vi "AddBandstoBandNames.vi"(11 "filter name":string) -> (1 "File Name":string[](array[string]), 3 "Extended Name":string[](array[string]))   [LabVIEW 2022 SP3]
uses:
  <vilib>/Utility/error.llb/whitespace.ctl
  <vilib>/Utility/error.llb/Trim Whitespace One-Sided.vi
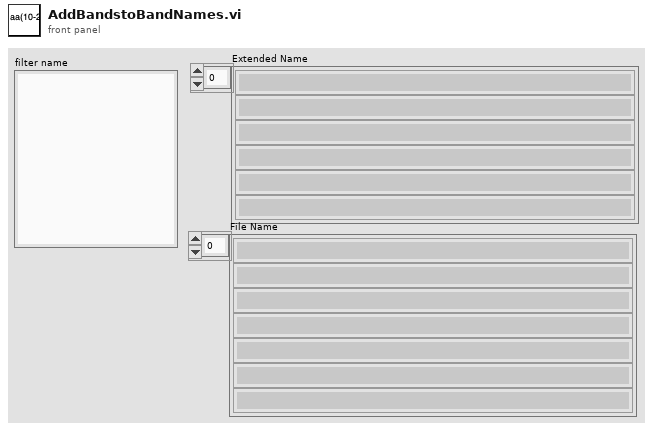
[diagram p1: front panel]
types:
  T1 = typedef "whitespace.ctl" = u16
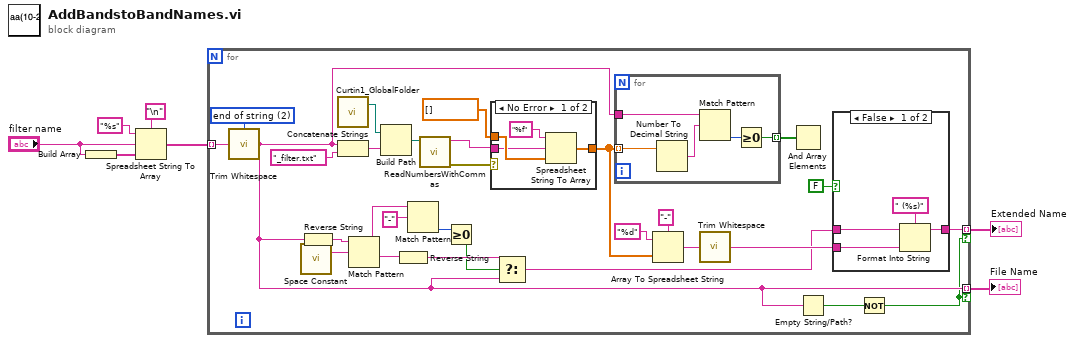
[diagram p0: block diagram]
diagram:
  n1 = Build Array("filter name") -> (w5:string[])
  n2 = Spreadsheet String To Array(delimiter (Tab)="\n" ("format string"), format string="%s", spreadsheet string="filter name", array type (2D Dbl)=w5) -> (array=w4:string[])
  n3 = for {
    tunnel: w4 -> [w25] mode=indexing
    tunnel: [w29] -> w3 mode=indexing if=w14
    tunnel: [w16] -> w2 mode=indexing if=w14
    w11 = T1 2 items=["both", "start of string", "end of string"] ("location (both)")
    n4 = call <vilib>:"Trim Whitespace.vi"("string"=w25, "location (both)"=w11) -> ("trimmed string"=w16:string)
    n5 = call <vilib>:"Space Constant.vi"() -> ("String"=w23:string)
    n6 = Reverse String(1:w16) -> (0:w24:string)
    n7 = call "Curtin1_GlobalFolder.vi"() -> ("LabVIEW Data Path"=w35:path)  [unwired: 1 in, 1 out]
    n8 = Concatenate Strings(w16, "_filter.txt" ("string")) -> (w36:string)
    n9 = Match Pattern(string=w24, regular expression=w23) -> (before substring=w13:string, after substring=w22:string)  [unwired: 1 in, 2 out]
    n10 = Build Path(base path=w35, name or relative path=w36) -> (appended path=w9:path)
    n11 = Reverse String(1:w22) -> (0:w20:string)
    n12 = Match Pattern(string=w13, regular expression="-" ("delimiter (Tab)")) -> (offset past match=w18:i32)  [unwired: 1 in, 3 out]
    n13 = call "ReadNumbersWithCommas.vi"("file (use dialog)"=w9) -> ("error out"=w10:errorcluster, "fixed"=w8:string)  [unwired: 7 in, 2 out]
    n14 = Greater Or Equal To 0?(x=w18) -> (x >= 0?=w17:bool)
    n15 = case shown="No Error" w10 {
      tunnel: [w48 w51] -> w26
      tunnel: w8 -> [w47 _]
      tunnel: dbl[] [] ("DataPath") -> [w50 w51]
      frame No Error {
        n16 = Spreadsheet String To Array(format string="%f", spreadsheet string=w47, array type (2D Dbl)=w50) -> (array=w48:dbl[])  [unwired: 1 in]
      }
      frame Error {
      }
    }
    n17 = Select(t=w20, s=w17, f=w16) -> (s? t:f=w19:string)
    n18 = for {
      tunnel: [w37] -> w28 mode=indexing
      tunnel: w16 -> [w40]
      tunnel: w26 -> [w39] mode=indexing
      n19 = Number To Decimal String(number=w39) -> (decimal integer string=w38:string)  [unwired: 1 in]
      n20 = Match Pattern(string=w40, regular expression=w38) -> (offset past match=w41:i32)  [unwired: 1 in, 3 out]
      n21 = Greater Or Equal To 0?(x=w41) -> (x >= 0?=w37:bool)
    }
    n22 = Array To Spreadsheet String(delimiter (Tab)="-", array=w26, 3:"%d" ("format string")) -> (spreadsheet string=w30:string)
    n23 = call <vilib>:"Trim Whitespace.vi"("string"=w30) -> ("trimmed string"=w27:string)  [unwired: 1 in]
    n24 = And Array Elements(Boolean array=w28) -> ()  [unwired: 1 out]
    n25 = Empty String/Path?(string/path=w16) -> (empty?=w15:bool)
    n26 = case shown="False" FALSE {
      tunnel: w19 -> [w44 w46]
      tunnel: [w43 w46] -> w29
      tunnel: w27 -> [w42 _]
      frame False {
        n27 = Format Into String(format string=" (%s)", initial string=w44, w42) -> (resulting string=w43:string)  [unwired: 1 in, 1 out]
      }
      frame True {
      }
    }
    n28 = Not(x=w15) -> (.not. x?=w14:bool)
  }
  "Extended Name" <- w3
  "File Name" <- w2
